vi "Level Eingabe pruefen.vi"(8 "aktueller PW-Level":i16, 10 "Passworte":T1) -> (2 "Passworte":T1)   [LabVIEW 2020, in "Passwort.lvlib"]
uses:
  Passwort.lvlib
  Passwort Array.ctl
  Passwort.ctl
  Visualisierungs Elemente/String - Eingabefeld.ctl
  Visualisierungs Elemente/Zahlen-Eingabefeld.ctl
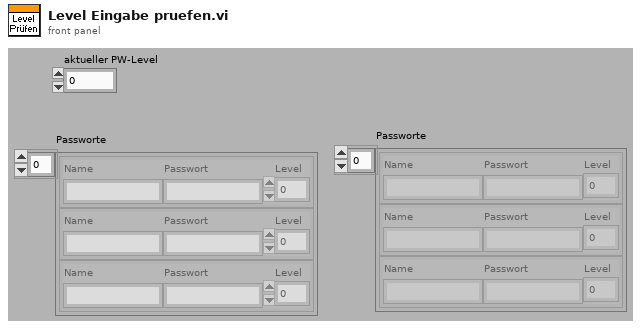
[diagram p1: front panel]
types:
  T1 = typedef "Passwort.lvlib/Passwort Array.ctl" = cluster{"Name":string, "Passwort":string, "Level":i16}[]
  T2 = typedef "Passwort.lvlib/Passwort.ctl" = cluster{"Name":T3, "Passwort":T3, "Level":T4}
  T3 = typedef "String - Eingabefeld.ctl" = string
  T4 = typedef "Zahlen-Eingabefeld.ctl" = sgl
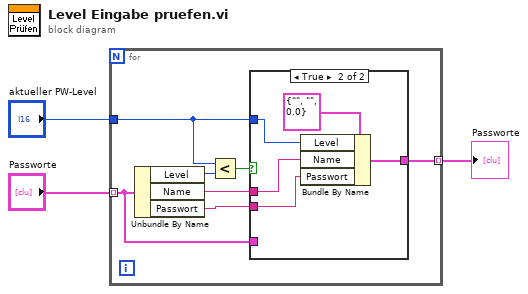
[diagram p0: block diagram]
diagram:
  n1 = for {
    tunnel: "Passworte" -> [w5] mode=indexing
    tunnel: "aktueller PW-Level" -> [w8]
    tunnel: [w4] -> w1 mode=indexing
    n2 = Unbundle By Name(w5) -> ("Level"=w10:i16, "Name"=w7:string, "Passwort"=w6:string)
    n3 = Less?(x=w8, y=w10) -> (x < y?=w9:bool)
    n4 = case shown="True" w9 {
      tunnel: w8 -> [_ w15]
      tunnel: w7 -> [_ w14]
      tunnel: w6 -> [_ w13]
      tunnel: w5 -> [w11 _]
      tunnel: [w11 w12] -> w4
      frame False {
      }
      frame True {
        n5 = Bundle By Name(cluster=T2 {"Name"="", "Passwort"="", "Level"=0.0} ("Passwort.lvlib:Passwort"), "Level"=w15, "Name"=w14, "Passwort"=w13) -> (w12:T2)
      }
    }
  }
  "Passworte" <- w1
